vi "Reverse2Darray -- SubVI.vi"(11 "Input Array":bool[][](array[boolean])=[[TRUE, FALSE, FALSE, FALSE], [TRUE, TRUE, FALSE, FALSE], [FALSE, TRUE, FALSE, FALSE], [FALSE, TRUE, TRUE, FALSE], [FALSE, FALSE, TRUE, FALSE], [FALSE, FALSE, TRUE, TRUE], [FALSE, FALSE, FALSE, TRUE], [TRUE, FALSE, FALSE, TRUE]]) -> (3 "Reverse Array":bool[][](array[boolean]))   [LabVIEW 2020]
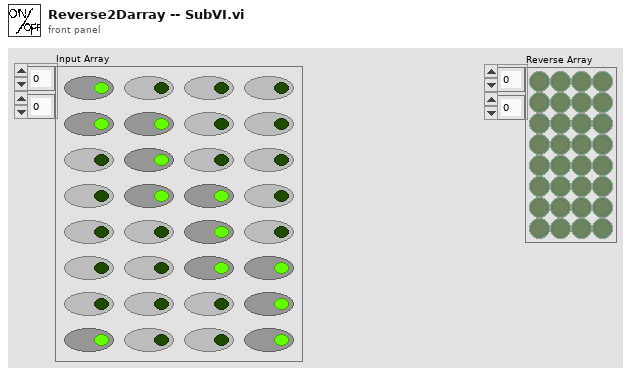
[diagram p1: front panel]
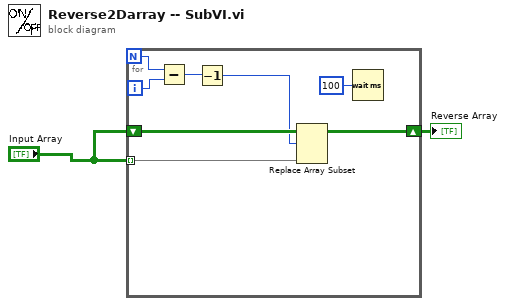
[diagram p0: block diagram]
diagram:
  n1 = for {
    N -> [w7]
    tunnel: "Input Array" -> [w4] mode=indexing
    shift-right: [w3] -> w1
    shift-left: "Input Array" -> [w9]
    i -> [w8]
    n2 = Subtract(x=w7, y=w8) -> (x-y=w6:i32)
    n3 = Decrement(x=w6) -> (x-1=w5:i32)
    n4 = Replace Array Subset "Replace Array Subset"(array=w9, new element=w4, index (row)=w5) -> (w3:bool[][])  [unwired: 1 in]
    n5 = Wait (ms)(milliseconds to wait=u32 100) -> ()  [unwired: 1 out]
  }
  "Reverse Array" <- w1
